vi "PH_Beckhoff.Read Database.vi"(2 "error in (no error)":errorcluster, 3 "DB Entry to read":string) -> (0 "error out":errorcluster, 1 "IP":string)   [LabVIEW 2014, in "PH_Beckhoff.lvlib"]
uses:
  PH_Beckhoff.lvlib
  PH_Common/PH_Common.lvlib
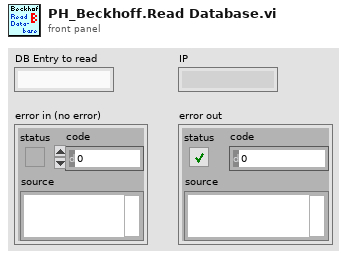
[diagram p1: front panel]
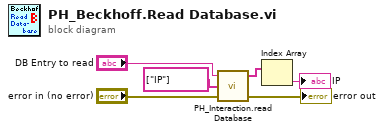
[diagram p0: block diagram]
diagram:
  n1 = call "PH_Interaction.read Database.vi"("error in (no error)"="error in (no error)", "Strings to search for"=string[] ["IP"] ("Strings to search for in"), "DB Entry to read"="DB Entry to read") -> ("error out"=→"error out":errorcluster, "Values"=w3:string[])  [unwired: 1 in]
  n2 = Index Array(array=w3) -> (element=→"IP":string)  [unwired: 1 in]
